vi "udp_publisher.vi"() -> ()   [LabVIEW 2014]
panel:
  in  "destination address":string
  in  "local port":u16
  in  "destination port or service name":u16
  out "error out":errorcluster
  in  "timeout ms (25000)":i32
  in  "data in":string
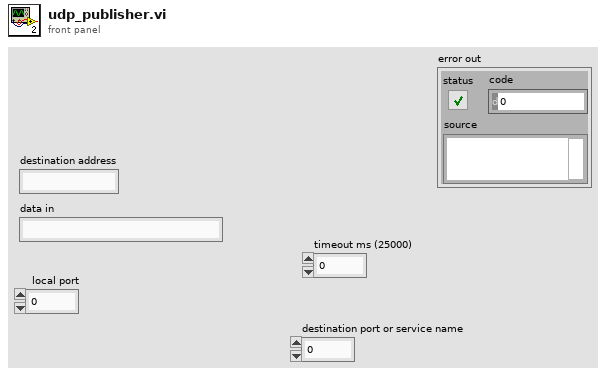
[diagram p1: front panel]
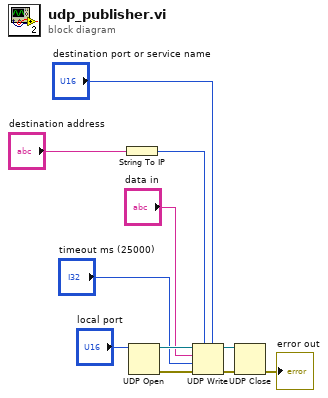
[diagram p0: block diagram]
diagram:
  n1 = String To IP(1:"destination address") -> (0:w2:u32)
  n2 = UDP Open(11:"local port") -> (port=w11:refnum<k16>, 0:w5:errorcluster)  [unwired: 4 in, 1 out]
  n3 = UDP Write(address=w2, port or service name="destination port or service name", connection ID=w11, data in="data in", 8:w5, 9:"timeout ms (25000)") -> (error out=w7:errorcluster, 3:w8:refnum<k16>)
  n4 = UDP Close(connection ID=w8, 8:w7) -> (error out=→"error out":errorcluster)  [unwired: 1 out]
